vi "Client Single Connection.vi"() -> ()   [LabVIEW 2021]
doc: "This WebSockets API example VI acts as a client to make an outgoing websockets connection. Receives/sends string data to the connected server."
uses:
  Reg/ctl/Y_short.ctl
  WebSockets/WebSocket/WebSocket.lvclass/WebSocket.ctl
  19e1ec6a-2dc8-4025-be8a-e5de19c8449a.vi
  WebSockets/WebSocket Client/WebSocket Client.lvclass
  D:/my_projects/projects/Algorithms/Labview/21/WebSockets/Source/WebSockets/WebSocket/WebSocket.lvclass
  <vilib>/JDP Science/JSONtext/JSON text to Variant.vi
  <vilib>/JDP Science/JSONtext/LVClass Serializer/JSONtext LVClass Serializer.lvclass
  WebSockets/WebSocket/WebSocket.lvclass
  Reg/control.lvlib
  <vilib>/JDP Science/JSONtext/JSONtext.lvlib
panel:
  out "Data out":T1={"Y_Source"=3, "Y_SetState"=0, "SP_Set"=0.0, "SP"=0.0, "PV"=0.0, "PV_State"={"code"=0, "visible"=FALSE, "color"=0}, "Y_preSet"=0.0, "Y_Set"=0.0, "Y"=0.0, "Y_State"={"code"=0, "visible"=FALSE, "color"=0}, "YB"=FALSE} {"Y" format="%.2f"; "Y_preSet" format="%.2f"; "SP" step=0.01 format="%.2f"; "Y_Set" format="%.2f"; "PV" step=0.01 format="%.2f"; "SP_Set" step=0.01 format="%.2f"}
  out "<JSON>":string[](array[string]) caption="<JSON>Items"
  out "Item Names":string[](array[string])
  in  "Disconnect":bool
  in  "Connect":bool
  in  "WebSockets URL":string="ws://echo.websocket.org"
  out "HTTP Headers":variant
  in  "Stop":bool
  out "Received Data":string
  in  "Send":bool
  in  "Data":string
  # "WebSockets Client Example"
  # "This VI is a simple example of sending/receiving data using WebSockets.\nIt opens a WebSockets Client connection to the WebSockets URL and can send / receive WebSockets data from the server.\n\nInstructions for use:\n1) Run this VI\n2) Enter the WebSockets URL that you wish to open a connection to (e.g. ws://echo.websocket.org) and click 'Connect'\n3) Enter text to send in 'Data' hit 'Send' to send to the WebSockets server\n4) WebSockets messages received from the server will be displayed in 'Received Data'"
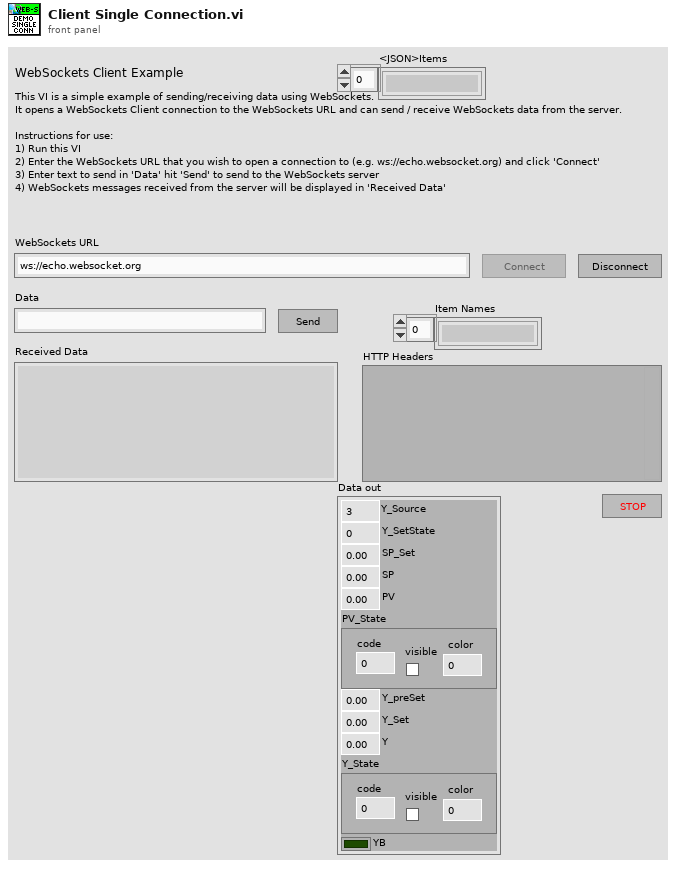
[diagram p1: front panel]
types:
  T1 = typedef "control.lvlib/Y_short.ctl" = cluster{"Y_Source":u8, "Y_SetState":u8, "SP_Set":dbl, "SP":dbl, "PV":dbl, "PV_State":cluster{"code":i32, "visible":bool, "color":u32}, "Y_preSet":dbl, "Y_Set":dbl, "Y":dbl, "Y_State":cluster{"code":i32, "visible":bool, "color":u32}, "YB":bool}
  T2 = enum8{"Enabled", "Disabled", "Disabled and Grayed Out"}
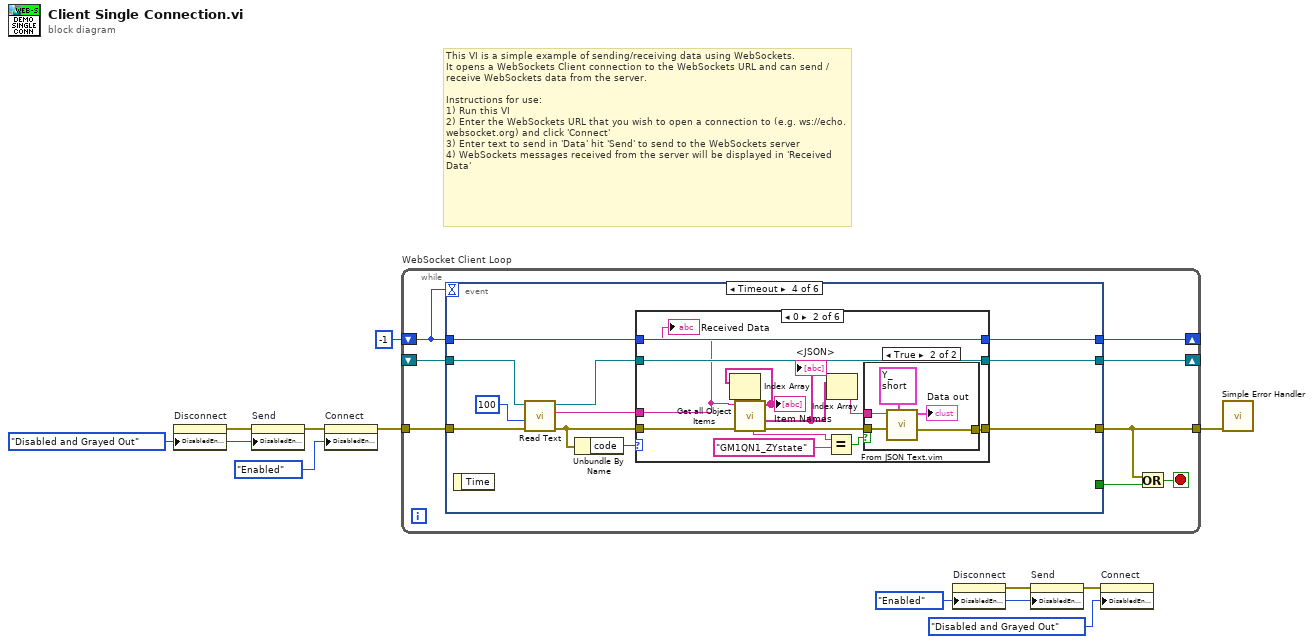
[diagram p0: block diagram]
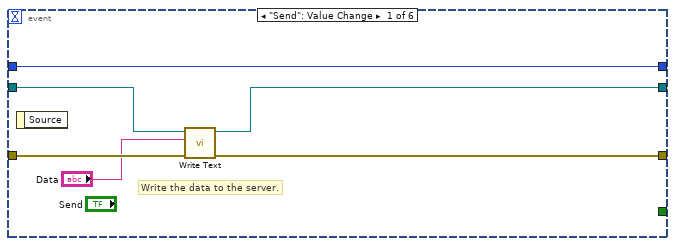
[diagram p2: hidden frame]
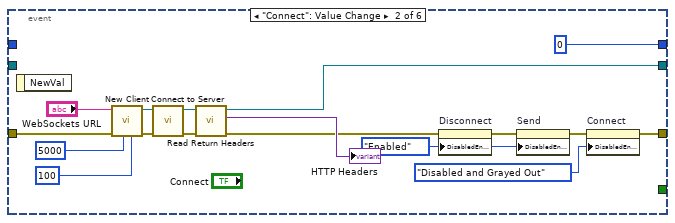
[diagram p3: hidden frame]
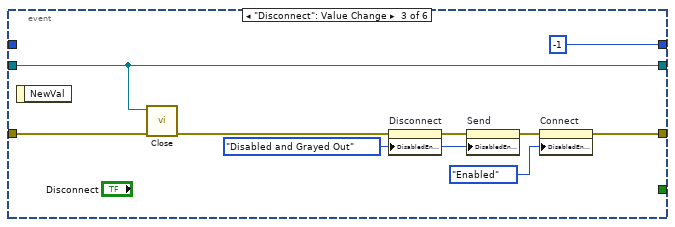
[diagram p4: hidden frame]
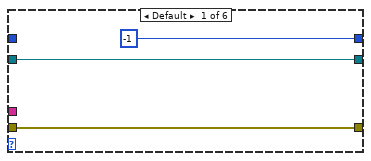
[diagram p5: hidden frame]
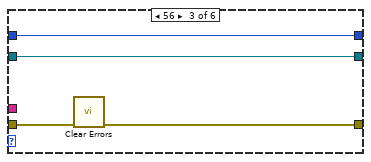
[diagram p7: hidden frame]
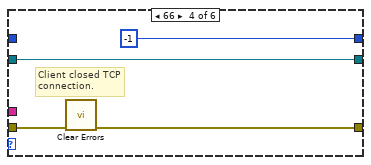
[diagram p8: hidden frame]
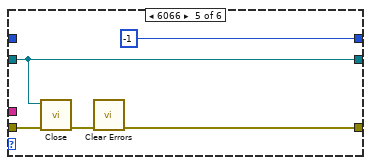
[diagram p9: hidden frame]
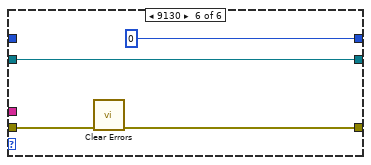
[diagram p10: hidden frame]
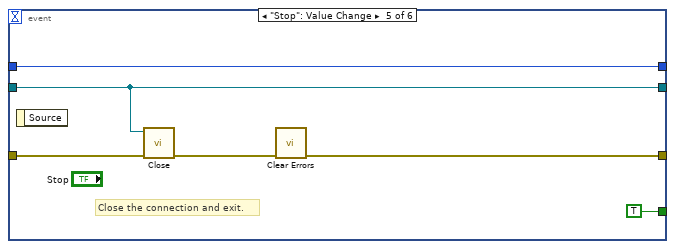
[diagram p11: hidden frame]
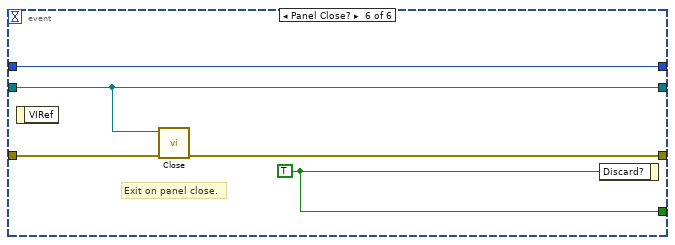
[diagram p12: hidden frame]
diagram:
  w4 = T2."Enabled" ("Disabled")
  w8 = T2."Disabled and Grayed Out" ("Disabled")
  # "This VI is a simple example of sending/receiving data using WebSockets.\nIt opens a WebSockets Client connection to the WebSockets URL and can send / receive WebSockets data from the server.\n\nInstructions for use:\n1) Run this VI\n2) Enter the WebSockets URL that you wish to open a connection to (e.g. ws://echo.websocket.org) and click 'Connect'\n3) Enter text to send in 'Data' hit 'Send' to send to the WebSockets server\n4) WebSockets messages received from the server will be displayed in 'Received Data'"
  n1 = property on="Disconnect" class="Bool"("DisabledEnum"=w8) -> (error out=w9:errorcluster)  [unwired: 2 in, 1 out]
  n2 = property on="Send" class="Bool"(error in=w9, "DisabledEnum"=w8) -> (error out=w3:errorcluster)  [unwired: 1 in, 1 out]
  n3 = property on="Connect" class="Bool"(error in=w3, "DisabledEnum"=T2."Enabled" ("Disabled")) -> (error out=w2:errorcluster)  [unwired: 1 in, 1 out]
  n4 = while "WebSocket Client Loop" {
    tunnel: [w16] -> w11
    tunnel: w2 -> [w19]
    shift-right: [w15] -> _
    shift-left: _ -> [w14]
    shift-right: [w13] -> _
    shift-left: -1 -> [w12]
    stop <- w17 stop-if-true
    n5 = event shown="[3] Timeout" {
      selector: _ -> [_ _ _ _ _ _]
      dyn-events: _ -> [_ _ _ _ _ _]
      timeout: w12 -> [_ _ _ _ _ _]
      tunnel: [_ _ _ _ TRUE w111] -> w18
      tunnel: [w24 w33 w43 w57 w104 w109] -> w16
      tunnel: w19 -> [w25 w42 w51 w62 w103 w110]
      tunnel: [w21 w40 w50 w54 w101 w108] -> w15
      tunnel: w14 -> [w22 _ w50 w61 w101 w108]
      tunnel: w12 -> [w20 _ _ w53 w105 w107]
      tunnel: [w20 0 -1 w52 w105 w107] -> w13
      event "Send": Value Change {
        # "Write the data to the server."
        n6 = event-data() -> ()  [unwired: 1 in, 1 out]
        n7 = call-dynamic "Write Text.vi"("error in (no error)"=w25, "String Data"="Data", "WebSocket in"=w22) -> ("error out"=w24:errorcluster, "WebSocket out"=w21:refnum<class "WebSocket.lvclass">)  [unwired: 7 in]
      }
      event "Connect": Value Change {
        w37 = T2."Enabled" ("Disabled")
        n8 = event-data() -> ()  [unwired: 1 in, 1 out]
        n9 = call "New Client.vi"("write operation timeout"=100 ("read operation timeout"), "read operation timeout"=5000 ("write operation timeout"), "error in (no error)"=w42, "WebSocket URL"="WebSockets URL") -> ("error out"=w28:errorcluster, "WebSocket Client out"=w29:refnum<class "WebSocket Client.lvclass">)  [unwired: 6 in]
        n10 = call "Connect to Server.vi"("error in (no error)"=w28, "WebSocket Client in"=w29) -> ("error out"=w26:errorcluster, "WebSocket Client out"=w27:refnum<class "WebSocket Client.lvclass">)  [unwired: 8 in]
        n11 = call "Read Return Headers.vi"("error in (no error)"=w26, "WebSocket in"=w27) -> ("error out"=w35:errorcluster, "Return Headers"=→"HTTP Headers":variant, "WebSocket out"=w40:refnum<class "WebSocket Client.lvclass">)  [unwired: 7 in]
        n12 = property on="Disconnect" class="Bool"(error in=w35, "DisabledEnum"=w37) -> (error out=w36:errorcluster)  [unwired: 1 in, 1 out]
        n13 = property on="Send" class="Bool"(error in=w36, "DisabledEnum"=w37) -> (error out=w34:errorcluster)  [unwired: 1 in, 1 out]
        n14 = property on="Connect" class="Bool"(error in=w34, "DisabledEnum"=T2."Disabled and Grayed Out" ("Disabled")) -> (error out=w33:errorcluster)  [unwired: 1 in, 1 out]
      }
      event "Disconnect": Value Change {
        w46 = T2."Disabled and Grayed Out" ("Disabled")
        n15 = event-data() -> ()  [unwired: 1 in, 1 out]
        n16 = call-dynamic "Close.vi"("error in (no error)"=w51, "WebSocket in"=w50) -> ("error out"=w44:errorcluster)  [unwired: 8 in, 1 out]
        n17 = property on="Disconnect" class="Bool"(error in=w44, "DisabledEnum"=w46) -> (error out=w45:errorcluster)  [unwired: 1 in, 1 out]
        n18 = property on="Send" class="Bool"(error in=w45, "DisabledEnum"=w46) -> (error out=w47:errorcluster)  [unwired: 1 in, 1 out]
        n19 = property on="Connect" class="Bool"(error in=w47, "DisabledEnum"=T2."Enabled" ("Disabled")) -> (error out=w43:errorcluster)  [unwired: 1 in, 1 out]
      }
      event Timeout {
        n20 = event-data() -> ()  [unwired: 1 in, 1 out]
        n21 = call-dynamic "Read Text.vi"("error in (no error)"=w62, "timeout ms (5000)"=100, "WebSocket in"=w61) -> ("error out"=w56:errorcluster, "Data"=w59:string, "WebSocket out"=w55:refnum<class "WebSocket.lvclass">)  [unwired: 6 in]
        n22 = Unbundle By Name(w56) -> ("code"=w58:i32)
        n23 = case shown="0" w58 {
          tunnel: w59 -> [_ w74 _ _ _ _]
          tunnel: [w65 w71 w86 w88 w92 w98] -> w57
          tunnel: w56 -> [w65 w75 w87 w91 w96 w97]
          tunnel: w55 -> [w64 w77 w85 w90 w94 w100]
          tunnel: [w64 w77 w85 w90 w94 w100] -> w54
          tunnel: w53 -> [_ w76 w84 _ _ _]
          tunnel: [-1 w76 w84 -1 -1 0] -> w52
          frame Default {
          }
          frame 0 {
            n24 = call <vilib>:"Get all Object Items.vi"("error in (no error)"=w75, "JSON"=w74) -> ("error out"=w73:errorcluster, "<JSON>"=w72:string[], "Item Names"=w67:string[])  [unwired: 6 in, 1 out]
            "Item Names" <- w67
            "<JSON>" <- w72
            n25 = Index Array(array=w67) -> (element=w66:string)  [unwired: 1 in]
            n26 = Equal?(x=w66, y="GM1QN1_ZYstate") -> (x = y?=w68:bool)
            n27 = Index Array(array=w72) -> (element=w70:string)  [unwired: 1 in]
            n28 = case shown="True" w68 {
              tunnel: w73 -> [w78 w82]
              tunnel: w70 -> [_ w81]
              tunnel: [w78 w80] -> w71
              frame False {
              }
              frame True {
                n29 = call "From JSON Text.vim"("Data Type and Default Value"=T1 {"Y_Source"=3, "Y_SetState"=0, "SP_Set"=0.0, "SP"=0.0, "PV"=0.0, "PV_State"={"code"=0, "visible"=FALSE, "color"=0}, "Y_preSet"=0.0, "Y_Set"=0.0, "Y"=0.0, "Y_State"={"code"=0, "visible"=FALSE, "color"=0}, "YB"=FALSE} ("Y_State"), "error in (no error)"=w82, "JSON"=w81) -> ("error out"=w80:errorcluster, "Data out"=→"Data out":T1)  [unwired: 7 in]
              }
            }
            "Received Data" <- w74
          }
          frame 56 {
            n30 = call <vilib>:"Clear Errors.vi"("error in (no error)"=w87) -> ("error out"=w86:errorcluster)  [unwired: 5 in, 1 out]
          }
          frame 66 {
            # "Client closed TCP connection."
            n31 = call <vilib>:"Clear Errors.vi"("error in (no error)"=w91) -> ("error out"=w88:errorcluster)  [unwired: 5 in, 1 out]
          }
          frame 6066 {
            n32 = call-dynamic "Close.vi"("error in (no error)"=w96, "WebSocket in"=w94) -> ("error out"=w95:errorcluster)  [unwired: 8 in, 1 out]
            n33 = call <vilib>:"Clear Errors.vi"("error in (no error)"=w95) -> ("error out"=w92:errorcluster)  [unwired: 5 in, 1 out]
          }
          frame 9130 {
            n34 = call <vilib>:"Clear Errors.vi"("error in (no error)"=w97) -> ("error out"=w98:errorcluster)  [unwired: 5 in, 1 out]
          }
        }
      }
      event "Stop": Value Change {
        # "Close the connection and exit."
        n35 = event-data() -> ()  [unwired: 1 in, 1 out]
        n36 = call-dynamic "Close.vi"("error in (no error)"=w103, "WebSocket in"=w101) -> ("error out"=w102:errorcluster)  [unwired: 8 in, 1 out]
        n37 = call <vilib>:"Clear Errors.vi"("error in (no error)"=w102) -> ("error out"=w104:errorcluster)  [unwired: 5 in, 1 out]
      }
      event Panel Close? {
        w111 = TRUE ("Discard?")
        # "Exit on panel close."
        n38 = event-data() -> ()  [unwired: 1 in, 1 out]
        n39 = call-dynamic "Close.vi"("error in (no error)"=w110, "WebSocket in"=w108) -> ("error out"=w109:errorcluster)  [unwired: 8 in, 1 out]
        n40 = event-data("Discard?"=w111) -> ()  [unwired: 1 in, 1 out]
      }
    }
    n41 = Or(x=w16, y=w18) -> (x .or. y?=w17:bool)
  }
  n42 = property on="Disconnect" class="Bool"("DisabledEnum"=w4) -> (error out=w5:errorcluster)  [unwired: 2 in, 1 out]
  n43 = property on="Send" class="Bool"(error in=w5, "DisabledEnum"=w4) -> (error out=w6:errorcluster)  [unwired: 1 in, 1 out]
  n44 = property on="Connect" class="Bool"(error in=w6, "DisabledEnum"=T2."Disabled and Grayed Out" ("Disabled")) -> ()  [unwired: 1 in, 2 out]
  n45 = call <vilib>:"Simple Error Handler.vi"("error in (no error)"=w11) -> ()  [unwired: 4 in, 5 out]
